vi "DeviceAttachedCallback.vi"(4 "User Parameter":variant, 5 "Event Data":cluster{"sender":refnum<k24>, "e":refnum<k24>}, 6 "Control Ref":refnum<k24>, 7 "Event Common Data":T1) -> ()   [LabVIEW 2020]
uses:
  System.Management
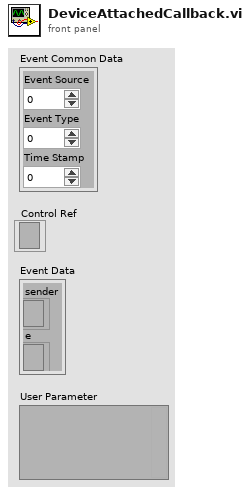
[diagram p1: front panel]
types:
  T1 = cluster{"Event Source":i32, "Event Type":u32, "Time Stamp":u32}
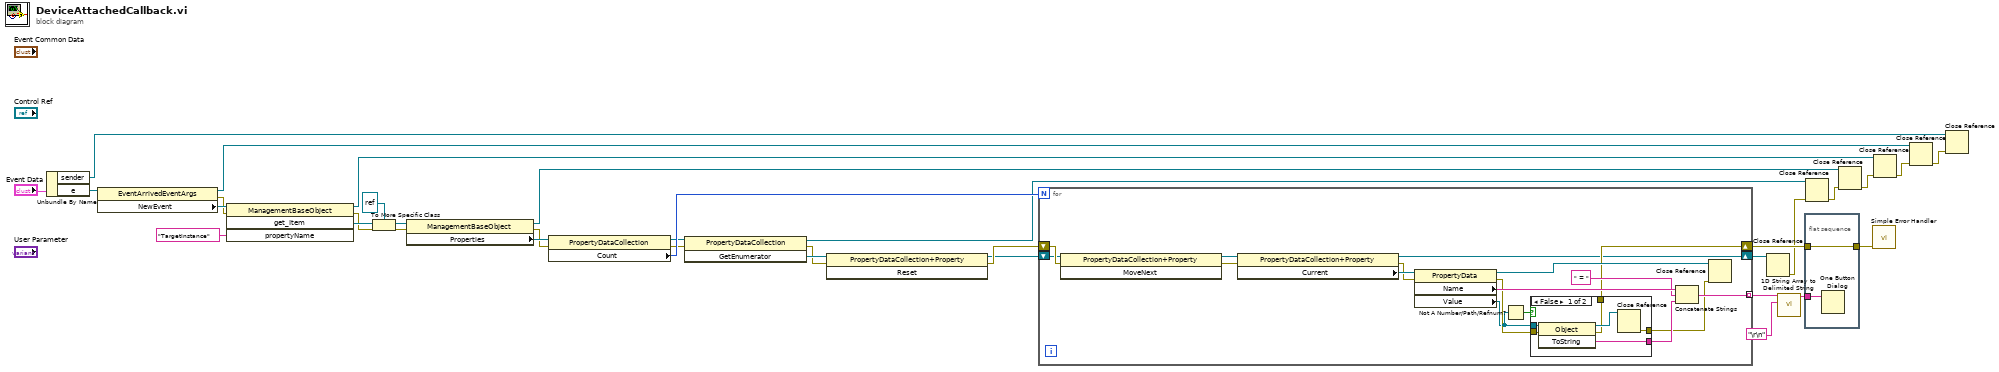
[diagram p0: block diagram]
diagram:
  n1 = Unbundle By Name("Event Data") -> ("sender"=w5:refnum<k24>, "e"=w34:refnum<k24>)
  n2 = property class="EventArrivedEventArgs"(reference=w34) -> (reference out=w7:refnum<k24>, error out=w25:errorcluster, "NewEvent"=w33:refnum<k24>)  [unwired: 1 in]
  n3 = invoke class="ManagementBaseObject" method="get_Item"(reference=w33, error in=w25, "propertyName"="TargetInstance") -> (reference out=w9:refnum<k24>, error out=w24:errorcluster, "get_Item"=w31:refnum<k24>)  [unwired: 1 in, 1 out]
  n4 = To More Specific Class(target class=refnum<k24> refnum, reference=w31, error in=w24) -> (specific class reference=w29:refnum<k24>, error out=w23:errorcluster)
  n5 = property class="ManagementBaseObject"(reference=w29, error in=w23) -> (reference out=w11:refnum<k24>, error out=w22:errorcluster, "Properties"=w28:refnum<k24>)
  n6 = property class="PropertyDataCollection"(reference=w28, error in=w22) -> (reference out=w26:refnum<k24>, error out=w21:errorcluster, "Count"=w27:i32)
  n7 = invoke class="PropertyDataCollection" method="GetEnumerator"(reference=w26, error in=w21) -> (reference out=w13:refnum<k24>, error out=w3:errorcluster, "GetEnumerator"=w4:refnum<k24>)  [unwired: 1 in]
  n8 = invoke class="PropertyDataCollection+Property" method="Reset"(reference=w4, error in=w3) -> (reference out=w1:refnum<k24>, error out=w2:errorcluster)  [unwired: 1 in, 1 out]
  n9 = for {
    N: w27 -> [_]
    shift-right: [w38] -> w15
    shift-left: w1 -> [w42]
    shift-right: [w39] -> w17
    shift-left: w2 -> [w43]
    tunnel: [w48] -> w20 mode=indexing
    n10 = invoke class="PropertyDataCollection+Property" method="MoveNext"(reference=w42, error in=w43) -> (reference out=w41:refnum<k24>, error out=w40:errorcluster)  [unwired: 1 in, 1 out]
    n11 = property class="PropertyDataCollection+Property"(reference=w41, error in=w40) -> (reference out=w38:refnum<k24>, error out=w45:errorcluster, "Current"=w52:refnum<k24>)
    n12 = property class="PropertyData"(reference=w52, error in=w45) -> (reference out=w46:refnum<k24>, error out=w44:errorcluster, "Name"=w51:string, "Value"=w36:refnum<k24>)
    n13 = Not A Number/Path/Refnum?(number/path/refnum=w36) -> (NaN/Path/Refnum?=w37:bool)
    n14 = case shown="False" w37 {
      tunnel: w36 -> [w58 _]
      tunnel: [w57 _] -> w50
      tunnel: [w55 _] -> w47
      tunnel: w44 -> [w54 w59]
      tunnel: [w53 w59] -> w39
      frame False {
        n15 = invoke class="Object" method="ToString"(reference=w58, error in=w54) -> (reference out=w56:refnum<k24>, error out=w53:errorcluster, "ToString"=w57:string)  [unwired: 1 in]
        n16 = Close Reference(reference=w56) -> (error out=w55:errorcluster)  [unwired: 1 in]
      }
      frame True {
      }
    }
    n17 = Concatenate Strings(w51, " = " ("string"), w50) -> (w48:string)
    n18 = Close Reference(reference=w46, error in (no error)=w47) -> ()  [unwired: 1 out]
  }
  n19 = Close Reference(reference=w15) -> (error out=w14:errorcluster)  [unwired: 1 in]
  n20 = call <vilib>:"1D String Array to Delimited String.vi"("delimiter"="\r\n", "string array"=w20) -> ("delimited string"=w18:string)  [unwired: 9 in]
  n21 = flat-sequence {
    tunnel: w18 -> [w61]
    tunnel: w17 -> [w60]
    tunnel: [w60] -> w16
    frame #0 {
      n22 = One Button Dialog(message=w61) -> ()  [unwired: 1 in, 1 out]
    }
  }
  n23 = Close Reference(reference=w13, error in (no error)=w14) -> (error out=w12:errorcluster)
  n24 = Close Reference(reference=w11, error in (no error)=w12) -> (error out=w10:errorcluster)
  n25 = call <vilib>:"Simple Error Handler.vi"("error in (no error)"=w16) -> ()  [unwired: 4 in, 5 out]
  n26 = Close Reference(reference=w9, error in (no error)=w10) -> (error out=w8:errorcluster)
  n27 = Close Reference(reference=w7, error in (no error)=w8) -> (error out=w6:errorcluster)
  n28 = Close Reference(reference=w5, error in (no error)=w6) -> ()  [unwired: 1 out]
